vi "Write Acyclic Tx Channel.vi"(6 "data with trigger in":T1[](array[typedef]), 8 "error in":errorcluster, 9 "labels settings for RT":T2[](array[typedef]) {"Label Timestamp Channel Data Reference" format="%.0x"; "Word Initial Raw Value" format="%032.0f"; "Label Disable/Trigger Channel Reference" format="%.0x"; "parameter driver data"."Tx parameter refs" format="%.0x"; "SDI" format="%02b"; "label" format="%.0o"}, 10 "channel number in":u8, 11 "board handle in":u8) -> (0 "error out":errorcluster, 2 "channel number out":u8, 3 "board handle out":u8)   [LabVIEW 2020, in "AIM ARINC 429 Hardware API.lvlib"]
uses:
  AIM ARINC 429 Hardware API.lvlib
  Shared/RT Label Settings.ctl
  Shared/Label.ctl
  Shared/RT Parameters.ctl
  Shared/Parameter Definition.ctl
  <vilib>/NI/NI VeriStand Encoding and Decoding/Encoding.ctl
  <vilib>/NI VeriStand/Custom Device API/Custom Device Item Ref.ctl
  Shared/Transfer Type.ctl
  <vilib>/NI VeriStand/Custom Device API/Data Reference.ctl
  Data Word with Trigger.ctl
  <instrlib>/AIM GmbH/_ARINC-429/subvi/Error Converter (ErrCode or Status).vi
  <instrlib>/AIM GmbH/_ARINC-429/subvi/Get Library Path.vi
  <instrlib>/AIM GmbH/_ARINC-429/VIs/Library/Api429Lib Error Desc Get.vi
  <instrlib>/AIM GmbH/_ARINC-429/subvi/Get Error Number Offset.vi
  <vilib>/Utility/error.llb/Error Cluster From Error Code.vi
  <instrlib>/AIM GmbH/_ARINC-429/AIM429LV.lvlib
  <vilib>/NI/NI VeriStand Encoding and Decoding/Encoding and Decoding.lvlib
  <vilib>/NI VeriStand/Custom Device API/Custom Device API.lvlib
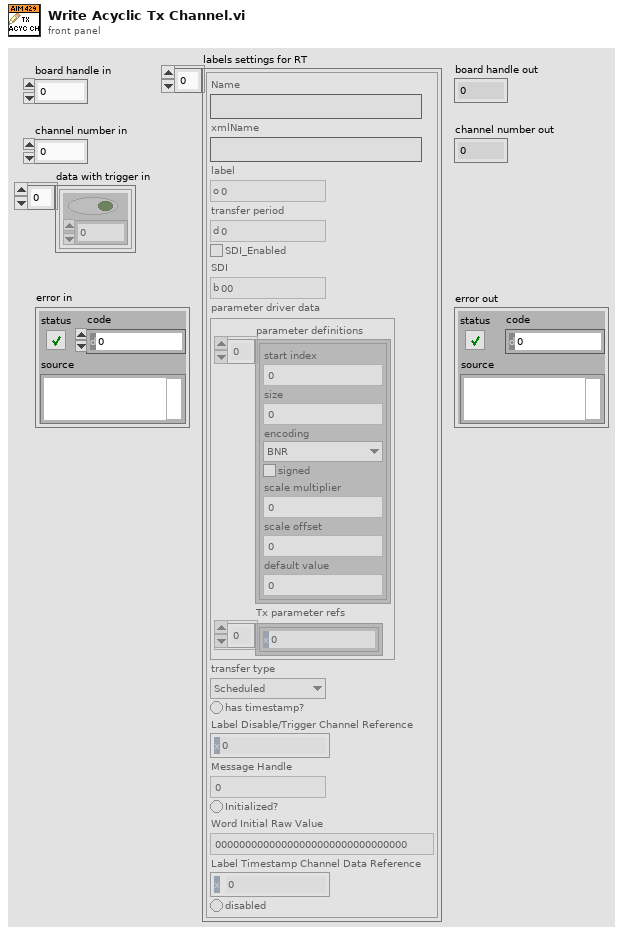
[diagram p1: front panel]
types:
  T1 = typedef "AIM ARINC 429 Hardware API.lvlib/Data Word with Trigger.ctl" = cluster{"Trigger":bool, "Data Word":u32}
  T2 = typedef "RT Label Settings.ctl" = cluster{"Name":string, "xmlName":string, "label":T3, "transfer period":u32, "SDI_Enabled":bool, "SDI":u8, "parameter driver data":T4, "transfer type":T8, "has timestamp?":bool, "Label Disable/Trigger Channel Reference":T7, "Message Handle":u64, "Initialized?":bool, "Word Initial Raw Value":u32, "Label Timestamp Channel Data Reference":T9, "disabled":bool}
  T3 = typedef "Label.ctl" = u8
  T4 = typedef "RT Parameters.ctl" = cluster{"parameter definitions":T5[], "Tx parameter refs":T7[]}
  T5 = typedef "Parameter Definition.ctl" = cluster{"start index":i32, "size":i32, "encoding":T6, "signed":bool, "scale multiplier":dbl, "scale offset":dbl, "default value":dbl}
  T6 = typedef "Encoding and Decoding.lvlib/Encoding.ctl" = enum16{"BNR", "BCD", "Discrete"}
  T7 = typedef "Custom Device API.lvlib/Custom Device Item Ref.ctl" = u64
  T8 = typedef "Transfer Type.ctl" = enum16{"Scheduled", "Acyclic", "Block", "Strobe"}
  T9 = typedef "Custom Device API.lvlib/Data Reference.ctl" = i32
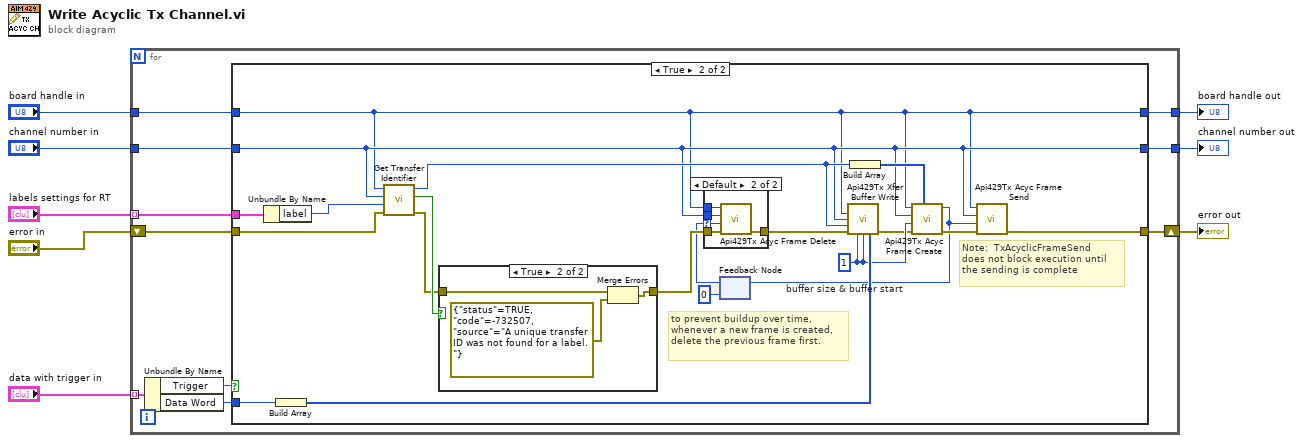
[diagram p0: block diagram]
diagram:
  n1 = for {
    tunnel: "board handle in" -> [w14]
    tunnel: "channel number in" -> [w15]
    tunnel: "labels settings for RT" -> [w18] mode=indexing
    shift-right: [w16] -> w3
    shift-left: "error in" -> [w17]
    tunnel: "data with trigger in" -> [w11] mode=indexing
    tunnel: [w13] -> w2
    tunnel: [w12] -> w1
    n2 = Unbundle By Name(w11) -> ("Trigger"=w9:bool, "Data Word"=w10:u32)
    n3 = case shown="True" w9 {
      tunnel: w18 -> [_ w41]
      tunnel: w17 -> [w21 w39]
      tunnel: w10 -> [_ w38]
      tunnel: [w21 w29] -> w16
      tunnel: w15 -> [w20 w23]
      tunnel: w14 -> [w19 w22]
      tunnel: [w20 w23] -> w13
      tunnel: [w19 w22] -> w12
      frame False {
        # "if no trigger was received for this label, do not write to the hardware"
      }
      frame True {
        w34 = u16 1  # buffer size & buffer start
        # "Note:  TxAcyclicFrameSend\ndoes not block execution until\nthe sending is complete"
        # "to prevent buildup over time, whenever a new frame is created, delete the previous frame first."
        n4 = Unbundle By Name(w41) -> ("label"=w40:T3)
        n5 = Build Array(w38) -> (w37:u32[])
        n6 = call "Get Transfer Identifier.vi"("error in"=w39, "label number in"=w40, "channel number in"=w23, "board number in"=w22) -> ("error out"=w35:errorcluster, "new entry created"=w36:bool, "Transfer ID out"=w33:u32)  [unwired: 5 in]
        n7 = case shown="True" w36 {
          tunnel: w35 -> [w48 w51]
          tunnel: [w48 w49] -> w27
          frame False {
          }
          frame True {
            n8 = Merge Errors(w51, errorcluster {"status"=TRUE, "code"=-732507, "source"="A unique transfer ID was not found for a label."} ("error constant")) -> (w49:errorcluster)
          }
        }
        n9 = feedback #1(u32 0 ("pulFrameId")) -> (w24:u32)
        n10 = case shown="Default" w24 {
          selector: w24 -> [_ w43]
          tunnel: [w42 w47] -> w28
          tunnel: w27 -> [w42 w46]
          tunnel: w23 -> [_ w45]
          tunnel: w22 -> [_ w44]
          frame 0 {
          }
          frame Default {
            n11 = call <instrlib>:"Api429Tx Acyc Frame Delete.vi"("error in (no error)"=w46, "ulFrameId"=w43, "ucChannel"=w45, "board_handle"=w44) -> ("error out"=w47:errorcluster)  [unwired: 7 in]
          }
        }
        n12 = call <instrlib>:"Api429Tx Xfer Buffer Write.vi"("board_handle"=w22, "b_Chn"=w23, "ul_XferId"=w33, "error in (no error)"=w28, "w_BufStart"=w34, "w_BufSize"=w34, "pl_LData"=w37) -> ("error out"=w31:errorcluster)  [unwired: 8 in]
        n13 = Build Array(w33) -> (w32:u32[])
        n14 = call <instrlib>:"Api429Tx Acyc Frame Create.vi"("pulXfers"=w32, "error in (no error)"=w31, "ulXferCnt"=w34, "ucChannel"=w23, "board_handle"=w22) -> ("error out"=w30:errorcluster, "pulFrameId"=w26:u32)  [unwired: 5 in]
        n15 = feedback-in #1(w26) -> ()
        n16 = call <instrlib>:"Api429Tx Acyc Frame Send.vi"("error in (no error)"=w30, "ulFrameId"=w26, "ucChannel"=w23, "board_handle"=w22) -> ("error out"=w29:errorcluster)  [unwired: 7 in]
      }
    }
  }
  "board handle out" <- w1
  "channel number out" <- w2
  "error out" <- w3
